vi "Bidireccional2.vi"() -> ()   [LabVIEW 2020]
uses:
  <vilib>/Instr/_visa.llb/VISA Configure Serial Port (Instr).vi
panel:
  in  "SW 6":bool
  in  "SW 7":bool
  in  "Stop Button":bool
  in  "SW 3":bool
  in  "SW 4":bool
  in  "SW 5":bool
  out "SW 8":bool
  in  "SW 2":bool
  in  "SW 1":bool
  out "ENVIO":string
  out "Escribir":bool
  in  "VISA resource name":refnum<visa-resource-name>
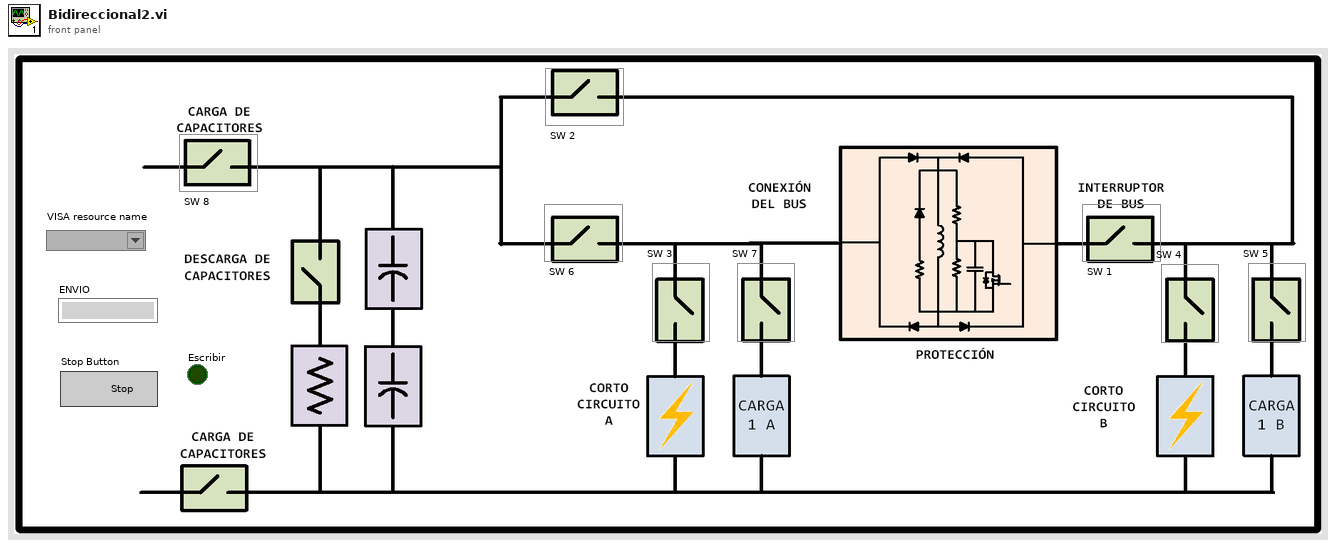
[diagram p1: front panel]
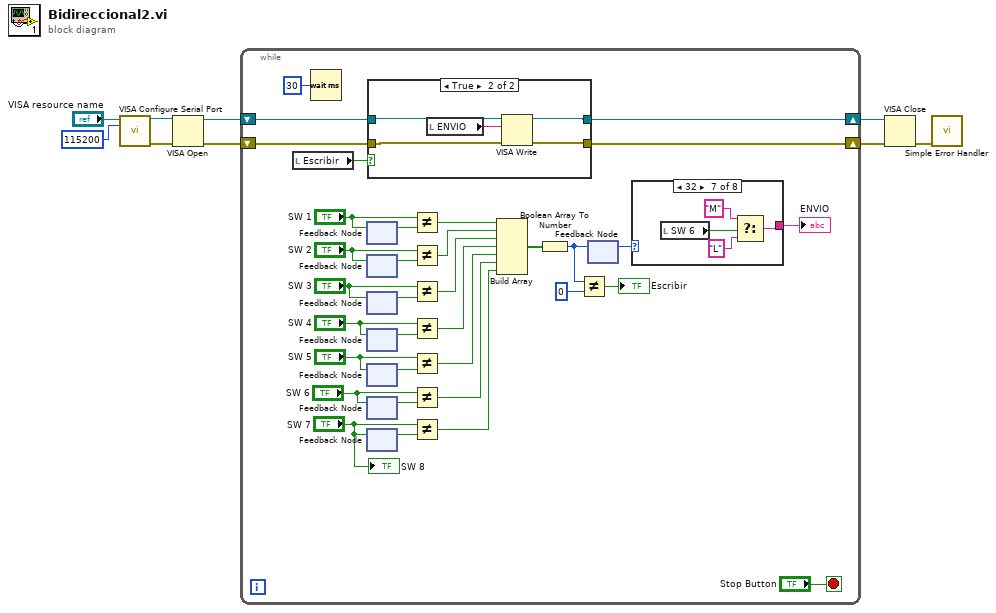
[diagram p0: block diagram]
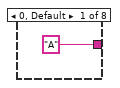
[diagram p2: hidden frame]
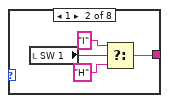
[diagram p3: hidden frame]
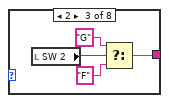
[diagram p4: hidden frame]
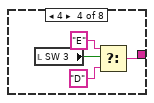
[diagram p5: hidden frame]
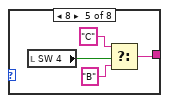
[diagram p6: hidden frame]
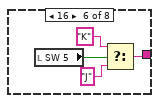
[diagram p7: hidden frame]
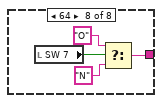
[diagram p8: hidden frame]
diagram:
  n1 = call-poly "VISA Configure Serial Port"("VISA resource name"="VISA resource name", "baud rate (9600)"=u32 115200) -> ("VISA resource name out"=w6:refnum<visa-resource-name>, "error out"=w7:errorcluster)  [unwired: 12 in]
  n2 = VISA Open(error in (no error)=w7, VISA resource name=w6) -> (VISA resource name=w5:refnum<visa-resource-name>, error out=w4:errorcluster)  [unwired: 3 in]
  n3 = while {
    shift-right: [w40] -> w2
    shift-left: w5 -> [w42]
    shift-right: [w39] -> w3
    shift-left: w4 -> [w41]
    stop <- "Stop Button" stop-if-true
    n4 = local read "Escribir"() -> (w38:bool)
    n5 = Wait (ms)(milliseconds to wait=u32 30) -> ()  [unwired: 1 out]
    n6 = feedback-in #1("SW 1") -> ()
    n7 = feedback #1() -> (w35:bool)  [unwired: 1 in]
    n8 = feedback #2() -> (w34:bool)  [unwired: 1 in]
    n9 = feedback-in #2("SW 2") -> ()
    n10 = feedback #3() -> (w29:bool)  [unwired: 1 in]
    n11 = feedback-in #3("SW 3") -> ()
    n12 = feedback #4() -> (w20:bool)  [unwired: 1 in]
    n13 = feedback-in #4("SW 4") -> ()
    n14 = feedback #5() -> (w17:bool)  [unwired: 1 in]
    n15 = feedback-in #5("SW 5") -> ()
    n16 = feedback #6() -> (w15:bool)  [unwired: 1 in]
    n17 = feedback-in #6("SW 6") -> ()
    n18 = feedback #7() -> (w13:bool)  [unwired: 1 in]
    n19 = feedback-in #7("SW 7") -> ()
    n20 = case shown="True" w38 {
      tunnel: [w74 w78] -> w40
      tunnel: w42 -> [w74 w76]
      tunnel: [w73 w79] -> w39
      tunnel: w41 -> [w73 w77]
      frame False {
      }
      frame True {
        n21 = local read "ENVIO"() -> (w75:string)
        n22 = VISA Write(VISA resource name=w76, write buffer=w75, error in (no error)=w77) -> (VISA resource name out=w78:refnum<visa-resource-name>, error out=w79:errorcluster)  [unwired: 1 out]
      }
    }
    n23 = Not Equal?(x="SW 1", y=w35) -> (x != y?=w28:bool)
    n24 = Not Equal?(x="SW 2", y=w34) -> (x != y?=w27:bool)
    n25 = Not Equal?(x="SW 3", y=w29) -> (x != y?=w26:bool)
    n26 = Not Equal?(x="SW 4", y=w20) -> (x != y?=w19:bool)
    n27 = Not Equal?(x="SW 5", y=w17) -> (x != y?=w16:bool)
    n28 = Not Equal?(x="SW 6", y=w15) -> (x != y?=w14:bool)
    n29 = Not Equal?(x="SW 7", y=w13) -> (x != y?=w12:bool)
    n30 = Build Array(w28, w27, w26, w19, w16, w14, w12) -> (w25:bool[])
    n31 = Boolean Array To Number(Boolean array=w25) -> (number=w24:u32)
    n32 = Not Equal?(x=w24, y=u32 0) -> (x != y?=→"Escribir":bool)
    n33 = feedback #8() -> (w31:u32)  [unwired: 1 in]
    n34 = feedback-in #8(w24) -> ()
    n35 = case shown="32" w31 {
      tunnel: ["A" ("element") w45 w50 w54 w59 w61 w65 w70] -> w32
      frame 0, Default {
      }
      frame 1 {
        n36 = local read "SW 1"() -> (w46:bool)
        n37 = Select(t="I" ("write buffer"), s=w46, f="H" ("write buffer")) -> (s? t:f=w45:string)
      }
      frame 2 {
        n38 = local read "SW 2"() -> (w49:bool)
        n39 = Select(t="G" ("element"), s=w49, f="F" ("element")) -> (s? t:f=w50:string)
      }
      frame 4 {
        n40 = local read "SW 3"() -> (w53:bool)
        n41 = Select(t="E" ("element"), s=w53, f="D" ("element")) -> (s? t:f=w54:string)
      }
      frame 8 {
        n42 = local read "SW 4"() -> (w57:bool)
        n43 = Select(t="C" ("element"), s=w57, f="B" ("element")) -> (s? t:f=w59:string)
      }
      frame 16 {
        n44 = local read "SW 5"() -> (w62:bool)
        n45 = Select(t="K" ("element"), s=w62, f="J" ("element")) -> (s? t:f=w61:string)
      }
      frame 32 {
        n46 = local read "SW 6"() -> (w66:bool)
        n47 = Select(t="M" ("element"), s=w66, f="L" ("element")) -> (s? t:f=w65:string)
      }
      frame 64 {
        n48 = local read "SW 7"() -> (w69:bool)
        n49 = Select(t="O" ("element"), s=w69, f="N" ("element")) -> (s? t:f=w70:string)
      }
    }
    "ENVIO" <- w32
    "SW 8" <- "SW 7"
  }
  n50 = VISA Close(VISA resource name=w2, error in (no error)=w3) -> (error out=w1:errorcluster)
  n51 = call <vilib>:"Simple Error Handler.vi"("error in (no error)"=w1) -> ()  [unwired: 4 in, 5 out]
